vi "OpenSensorProtocol.vi"(0 "Baud Rate":u32=9600, 1 "Timeout Value (ms)":u32=5000, 2 "Termination Char (0xA = '\\n' = LF)":u8=10, 3 "Enable Termination Char? (T)":bool=TRUE, 5 "Data Bits":u16=8, 7 "Parity":u16(ring) items=["None", "Odd", "Even", "Mark", "Space"], 9 "Stop Bits":u16(ring)=10 items=["1.0"=10, "1.5"=15, "2.0"=20], 12 "Flow Control":u16(ring) items=["None", "XON/XOFF", "RTS/CTS", "XON/XOFF & RTS/CTS", "DTR/DSR", "XON/XOFF & DTR/DSR"], 13 "Serial Port":T2) -> (4 "SerialPortRef":T1)   [LabVIEW 2014]
uses:
  <vilib>/Rock Robotics/WPI/SerialPort/WPI_SerialPort.ctl
  <vilib>/Rock Robotics/WPI/SerialPort/WPI_SerialPortRef.ctl
  Global Data.vi
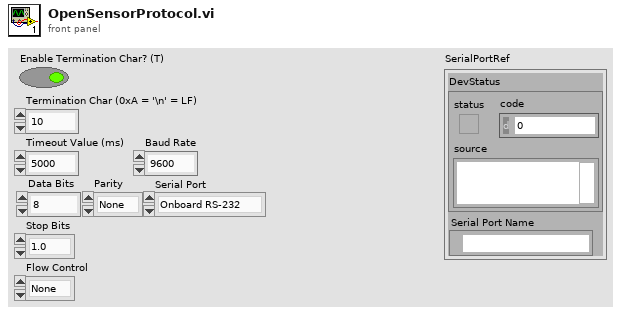
[diagram p1: front panel]
types:
  T1 = typedef "WPI_SerialPortRef.ctl" = cluster{"DevStatus":errorcluster, "Serial Port Name":refnum<visa-resource-name>}
  T2 = typedef "WPI_SerialPort.ctl" = enum16{"Onboard RS-232", "MXP TTL"}
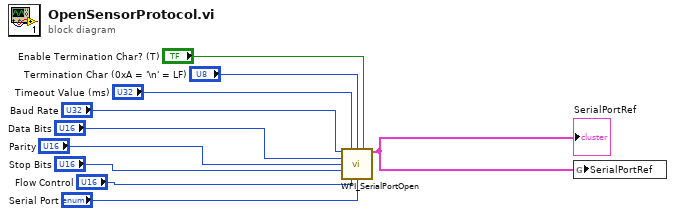
[diagram p0: block diagram]
diagram:
  n1 = call <vilib>:"WPI_SerialPortOpen.vi"("Baud Rate"="Baud Rate", "Timeout Value (ms)"="Timeout Value (ms)", "Termination Char (0xA = '\\n' = LF)"="Termination Char (0xA = '\\n' = LF)", "Enable Termination Char? (T)"="Enable Termination Char? (T)", "Data Bits"="Data Bits", "Parity"="Parity", "Stop Bits"="Stop Bits", "Flow Control"="Flow Control", "Serial Port"="Serial Port") -> ("SerialPortRef"=w1:T1)  [unwired: 5 in, 1 out]
  "SerialPortRef" <- w1
  n2 = global write "Global Data.vi" "SerialPortRef"(w1) -> ()
